vi "Globals_Real.vi"() -> ()   [LabVIEW 2014]
panel:
  out "Angular Rate Graph":dbl[][](graph)
  out "Angular Displacement Graph":dbl[][](graph)
  in  "Ind 2":dbl
  in  "Len":dbl
  out "Linear Acceleration":dbl[](array[numeric])
  out "Angular Displacement (Gyro)":dbl[](array[numeric])
  out "Angular Gyro Rate [LSB/sec":dbl[](array[numeric])
  out "Temperature":dbl
  in  "Ts":dbl=1000.0
  in  "Reset Integrator":bool
  in  "stop":bool
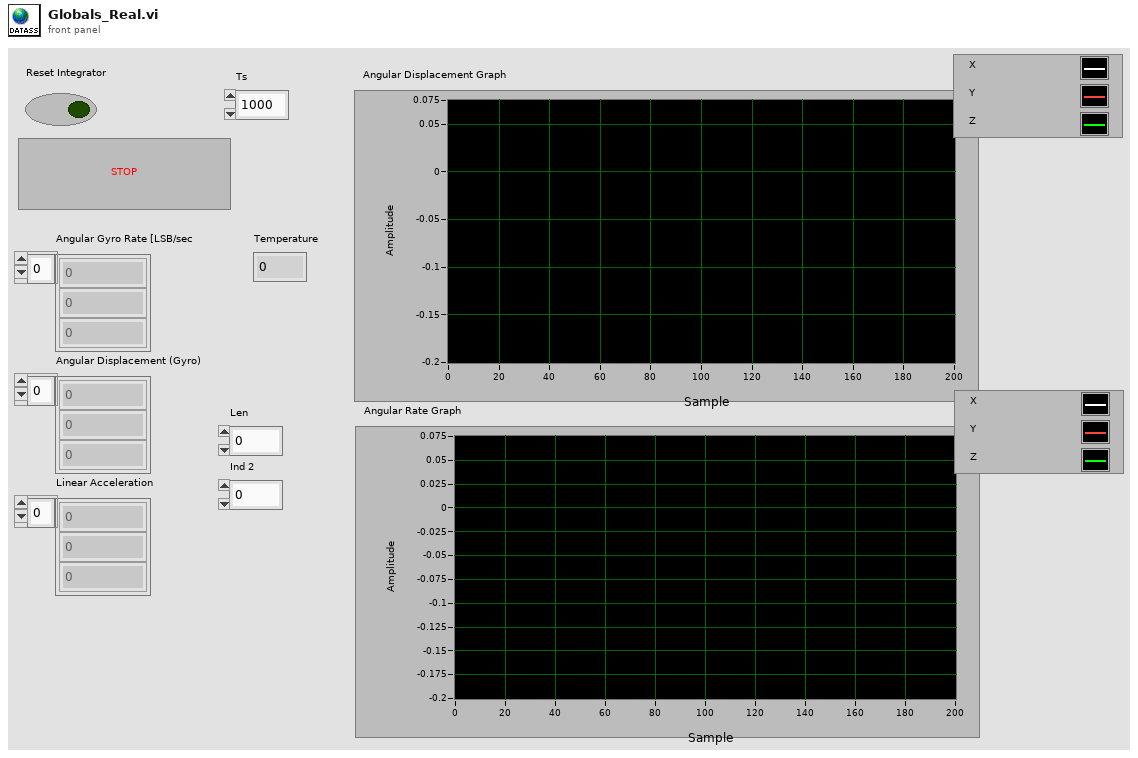
[diagram p1: front panel]
diagram:
